vi "RunAllScripts.vi"(8 "ErrorArray":errorcluster[](array[cluster])) -> (0 "ErrorArray":errorcluster[](array[cluster]))   [LabVIEW 2018]
uses:
  clUserEventDataType.ctl
  <vilib>/event_ctls.llb/usereventprio.ctl
  <userlib>/NIST/NISTErrorLib/NISTErrorLib.lvlib
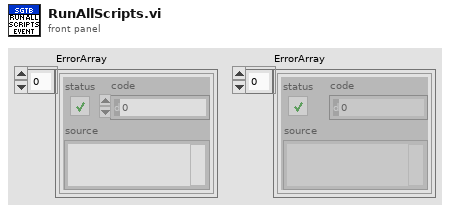
[diagram p1: front panel]
types:
  T1 = typedef "usereventprio.ctl" = enum32{"high priority", "normal priority"}
  T2 = typedef "clUserEventDataType.ctl" = cluster{"Data":variant}
  T3 = typedef "clUserEvents.ctl" = cluster{"StopEvent":refnum<user-event>, "RefreshUserEvents":refnum<user-event>, "StatusUpdate":refnum<user-event>, "RunAllScripts":refnum<user-event>}
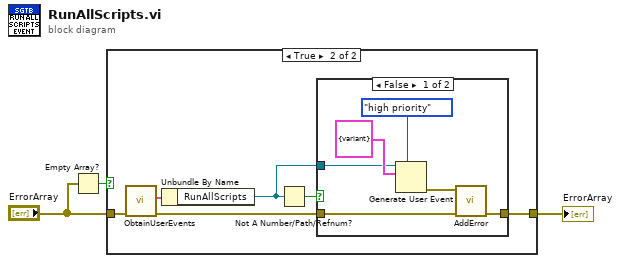
[diagram p0: block diagram]
diagram:
  n1 = Empty Array?(array="ErrorArray") -> (empty?=w3:bool)
  n2 = case shown="True" w3 {
    tunnel: "ErrorArray" -> [w4 w6]
    tunnel: [w4 w5] -> w1
    frame False {
    }
    frame True {
      n3 = call "ObtainUserEvents.vi"("ErrorArray"=w6) -> ("ErrorArray"=w8:errorcluster[], "clUserEvents"=w10:T3)  [unwired: 9 in]
      n4 = Unbundle By Name(w10) -> ("RunAllScripts"=w7:refnum<user-event>)
      n5 = Not A Number/Path/Refnum?(number/path/refnum=w7) -> (NaN/Path/Refnum?=w9:bool)
      n6 = case shown="False" w9 {
        tunnel: w8 -> [w14 w17]
        tunnel: w7 -> [w15 _]
        tunnel: [w11 w17] -> w5
        frame False {
          n7 = Generate User Event(priority (normal)=usereventprio."high priority", user event=w15, event data cluster=T2 {"Data"=variant} ("clUserEventData")) -> (error out=w13:errorcluster)  [unwired: 1 in, 1 out]
          n8 = call <userlib>:"AddError.vi"("ErrorArray In"=w14, "error in (no error)"=w13) -> ("ErrorArray Out"=w11:errorcluster[])  [unwired: 8 in, 1 out]
        }
        frame True {
        }
      }
    }
  }
  "ErrorArray" <- w1
